vi "Install CIN.vi"   [LabVIEW 2012]
doc: "Helps install the appropriate CIN. This will have to do until the conditional compile structure actually works on all platforms."
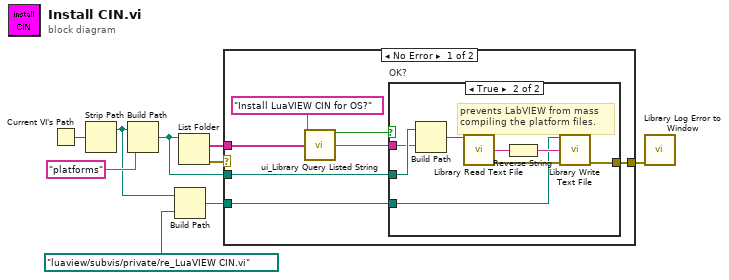
[diagram p0: block diagram]
diagram:
  n1 = Current VI's Path() -> (path=w9:path)
  n2 = Strip Path(path=w9) -> (stripped path=w2:path)  [unwired: 1 out]
  n3 = Build Path(base path=w2, name or relative path="platforms") -> (appended path=w4:path)
  n4 = Build Path(base path=w2, name or relative path=path "luaview/subvis/private/re_LuaVIEW CIN.vi") -> (appended path=w1:path)
  n5 = List Folder(path=w4) -> (filenames=w5:string[], error out=w7:errorcluster)  [unwired: 3 in, 2 out]
  n6 = case shown="No Error" w7 {
    selector: w7 -> [_ w25]
    tunnel: [w11 w25] -> w6
    tunnel: w5 -> [w16 _]
    tunnel: w4 -> [w12 _]
    tunnel: w1 -> [w10 _]
    frame No Error {
      n7 = call "ui_Library Query Listed String.vi"("prompt"="Install LuaVIEW CIN for OS?", "list of strings"=w16) -> ("OKed?"=w14:bool, "selected string"=w13:string)  [unwired: 12 in]
      n8 = case "OK?" shown="True" w14 {
        tunnel: w13 -> [_ w23]
        tunnel: w12 -> [_ w24]
        tunnel: [_ w21] -> w11
        tunnel: w10 -> [_ w17]
        frame False {
        }
        frame True {
          # "prevents LabVIEW from mass\ncompiling the platform files."
          n9 = Build Path(base path=w24, name or relative path=w23) -> (appended path=w22:path)
          n10 = call "Library Read Text File.vi"("file path"=w22) -> ("read text"=w19:string, "error out"=w20:errorcluster)  [unwired: 12 in, 1 out]
          n11 = Reverse String(1:w19) -> (0:w18:string)
          n12 = call "Library Write Text File.vi"("file path"=w17, "text to write"=w18, "error in (no error)"=w20) -> ("error out"=w21:errorcluster)  [unwired: 11 in, 1 out]
        }
      }
    }
    frame Error {
    }
  }
  n13 = call "Library Log Error to Window.vi"("error in (no error)"=w6) -> ()  [unwired: 13 in, 2 out]
